vi "AlazarGetBoardBySystemHandle.vi"(0 "Sys Handle":u64, 1 "Board ID":u32, 2 "error in (no error)":errorcluster) -> (3 "Sys Handle":u64, 4 "Board Handle":u64, 5 "Return Code":u32, 6 "error out":errorcluster)   [LabVIEW 2009]
doc: "Get a handle to a board in a board system where the board system is specified by a handle to its master board, and the board by its identifier within the board system."
uses:
  ATSApi.dll
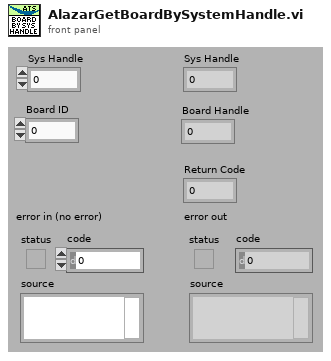
[diagram p1: front panel]
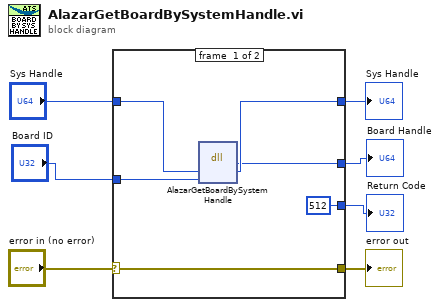
[diagram p0: block diagram]
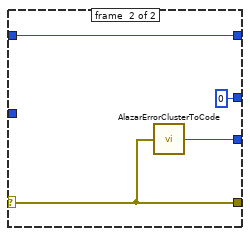
[diagram p2: hidden frame]
diagram:
  n1 = case shown="No Error" "error in (no error)" {
    selector: "error in (no error)" -> [w11 w17]
    tunnel: [w11 w17] -> w6
    tunnel: [u32 512 w16] -> w5
    tunnel: "Sys Handle" -> [w13 w15]
    tunnel: [w12 w15] -> w3
    tunnel: "Board ID" -> [w9 _]
    tunnel: [w8 u32 0] -> w1
    frame #0 {
      n2 = dll-call lib="ATSApi.dll" fn="AlazarGetBoardBySystemHandle"("handle"=w13, "boardId"=w9) -> ("return type"=w8:u64, "handle"=w12:u64)  [unwired: 4 in, 2 out]
    }
    frame #1 {
      n3 = call "AlazarErrorClusterToCode.vi"("error in (no error)"=w17) -> ("Error Code"=w16:u32)
    }
  }
  "Sys Handle" <- w3
  "error out" <- w6
  "Return Code" <- w5
  "Board Handle" <- w1
